vi "GFITS_GetDatesFmList.vi"(9 "List In":string[][](table), 10 "action":string, 11 "timestamp":string) -> (1 "List Out":string[][](table))   [LabVIEW 2016]
panel:
  out "timestamp 2":string
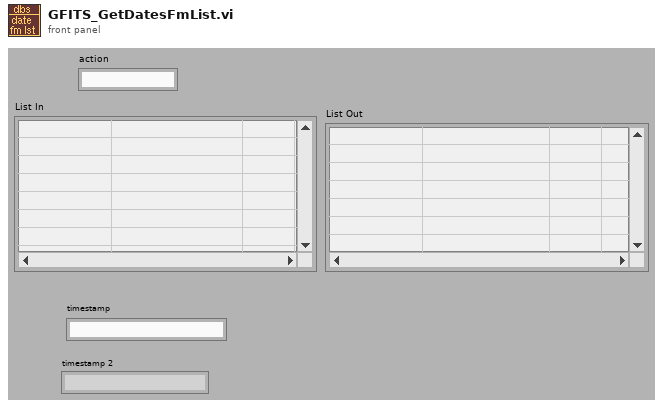
[diagram p1: front panel]
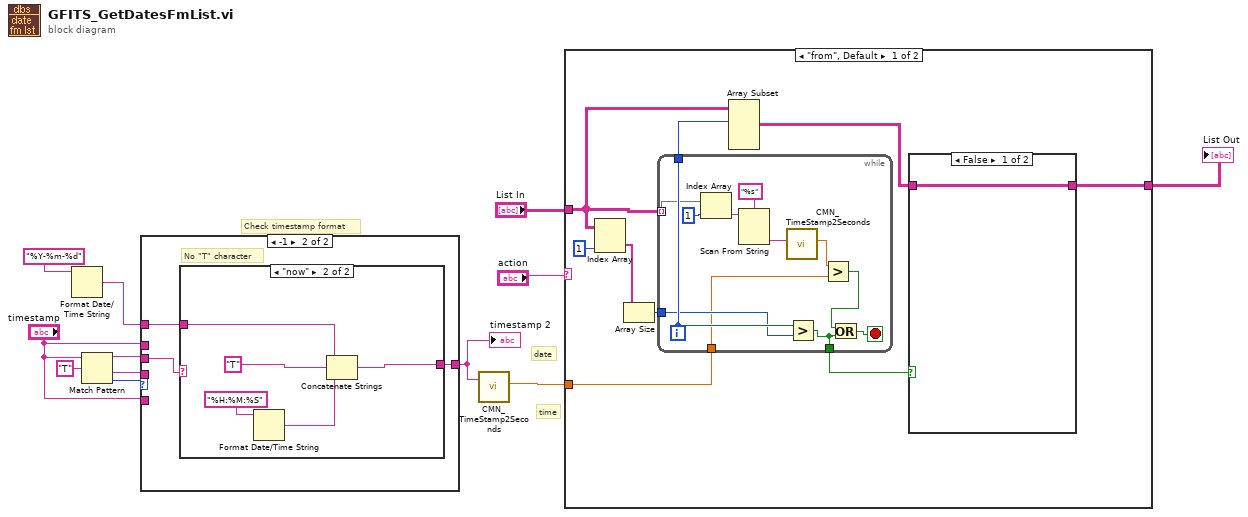
[diagram p0: block diagram]
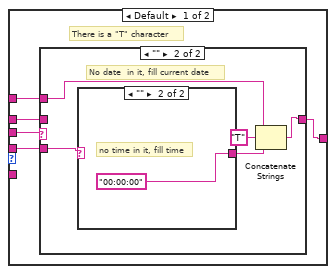
[diagram p2: hidden frame]
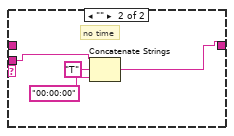
[diagram p4: hidden frame]
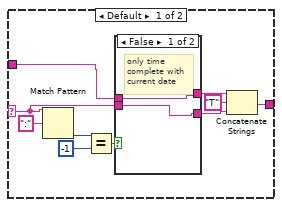
[diagram p6: hidden frame]
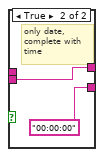
[diagram p7: hidden frame]
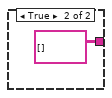
[diagram p8: hidden frame]
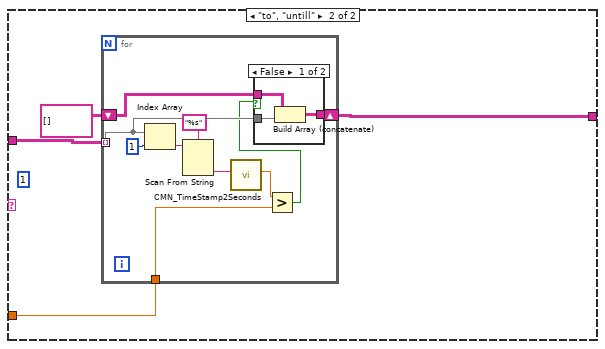
[diagram p9: hidden frame]
diagram:
  # "Check timestamp format"
  # "time"
  # "date"
  n1 = Format Date/Time String(time format string (%c)="%Y-%m-%d") -> (date/time string=w2:string)  [unwired: 2 out]
  n2 = Match Pattern(string="timestamp", regular expression="T") -> (before substring=w9:string, after substring=w8:string, offset past match=w5:i32)  [unwired: 2 out]
  n3 = case shown="-1" w5 {
    tunnel: w9 -> [w17 w36]
    tunnel: w8 -> [w15 _]
    tunnel: "timestamp" -> [_ _]
    tunnel: "timestamp" -> [w14 _]
    tunnel: w2 -> [w16 w35]
    tunnel: [w13 w34] -> w1
    frame Default {
      # "There is a \"T\" character"
      n4 = case shown="\"\"" w17 {
        selector: w17 -> [w18 _]
        tunnel: w16 -> [_ w28]
        tunnel: w15 -> [w21 w31]
        tunnel: w14 -> [w20 _]
        tunnel: [w19 w27] -> w13
        frame Default {
          # "date is there"
          n5 = case shown="Default" w21 {
            tunnel: w20 -> [w22 _]
            tunnel: [w22 w23] -> w19
            tunnel: w18 -> [_ w25]
            frame Default {
              # "time is there"
            }
            frame "" {
              # "no time"
              n6 = Concatenate Strings(w25, "T" ("string"), "00:00:00" ("string")) -> (w23:string)
            }
          }
        }
        frame "" {
          # "No date  in it, fill current date"
          n7 = case shown="\"\"" w31 {
            selector: w31 -> [w32 _]
            tunnel: [w32 "00:00:00" ("string")] -> w29
            frame Default {
            }
            frame "" {
              # "no time in it, fill time"
            }
          }
          n8 = Concatenate Strings(w28, "T" ("string"), w29) -> (w27:string)
        }
      }
    }
    frame -1 {
      # "No \"T\" character"
      n9 = case shown="\"now\"" w36 {
        selector: w36 -> [w38 _]
        tunnel: w35 -> [w40 w55]
        tunnel: [w42 w53] -> w34
        frame Default {
          n10 = Match Pattern(string=w38, regular expression=":") -> (offset past match=w45:i32)  [unwired: 4 out]
          n11 = Equal?(x=w45, y=-1) -> (x = y?=w41:bool)
          n12 = case shown="False" w41 {
            tunnel: w40 -> [w47 _]
            tunnel: [w48 "00:00:00"] -> w39
            tunnel: w38 -> [w48 w49]
            tunnel: [w47 w49] -> w37
            frame False {
              # "only time\ncomplete with\ncurrent date"
            }
            frame True {
              # "only date, \ncomplete with \ntime"
            }
          }
          n13 = Concatenate Strings(w37, "T" ("string"), w39) -> (w42:string)
        }
        frame "now" {
          n14 = Format Date/Time String(time format string (%c)="%H:%M:%S") -> (date/time string=w51:string)  [unwired: 2 out]
          n15 = Concatenate Strings(w55, "T" ("string"), w51) -> (w53:string)
        }
      }
    }
  }
  "timestamp 2" <- w1
  n16 = call "CMN_TimeStamp2Seconds.vi"("TimeStamp string (yyyy-mm-ddThh:mm:ss)"=w1) -> ("seconds out"=w7:dbl)  [unwired: 1 in, 8 out]
  n17 = case shown="\"from\", Default" "action" {
    tunnel: "List In" -> [w60 w82]
    tunnel: w7 -> [w57 w81]
    tunnel: [w56 w80] -> w6
    frame "from", Default {
      n18 = Index Array(array=w60, index (col)=1 ("disabled index (col)")) -> (element=w63:string[])  [unwired: 1 in]
      n19 = Array Size(array=w63) -> (size(s)=w62:i32)
      n20 = while {
        tunnel: w60 -> [w71] mode=indexing
        tunnel: w62 -> [w73]
        tunnel: [w72] -> w61
        tunnel: [w74] -> w59
        tunnel: w57 -> [w68]
        i -> [w74]
        stop <- w75 stop-if-true
        n21 = Index Array(array=w71, index=1) -> (element=w77:string)
        n22 = Scan From String(format string="%s", input string=w77) -> (output 1=w70:string)  [unwired: 2 in, 4 out]
        n23 = call "CMN_TimeStamp2Seconds.vi"("TimeStamp string (yyyy-mm-ddThh:mm:ss)"=w70) -> ("seconds out"=w69:dbl)  [unwired: 1 in, 8 out]
        n24 = Greater?(x=w74, y=w73) -> (0:w72:bool)
        n25 = Greater?(x=w69, y=w68) -> (0:w67:bool)
        n26 = Or(x=w67, y=w72) -> (x .or. y?=w75:bool)
      }
      n27 = Array Subset(array=w60, index (row)=w59) -> (w58:string[][])  [unwired: 3 in]
      n28 = case shown="False" w61 {
        tunnel: w58 -> [w65 _]
        tunnel: [w65 string[][] []] -> w56
        frame False {
        }
        frame True {
        }
      }
    }
    frame "to", "untill" {
      (unwired) 1 ("disabled index (col)")
      n29 = for {
        tunnel: w82 -> [w86] mode=indexing
        tunnel: w81 -> [w87]
        shift-right: [w84] -> w80
        shift-left: string[][] [] -> [w83]
        n30 = Index Array(array=w86, index=1) -> (element=w91:string)
        n31 = Scan From String(format string="%s", input string=w91) -> (output 1=w89:string)  [unwired: 2 in, 4 out]
        n32 = call "CMN_TimeStamp2Seconds.vi"("TimeStamp string (yyyy-mm-ddThh:mm:ss)"=w89) -> ("seconds out"=w88:dbl)  [unwired: 1 in, 8 out]
        n33 = Greater?(x=w88, y=w87) -> (0:w85:bool)
        n34 = case shown="False" w85 {
          tunnel: w86 -> [w95 _]
          tunnel: [w94 w96] -> w84
          tunnel: w83 -> [w93 w96]
          frame False {
            n35 = Build Array (concatenate)(w93, w95) -> (w94:string[][])
          }
          frame True {
          }
        }
      }
    }
  }
  "List Out" <- w6
